vi "amplitude modulation and demodulation.vi"() -> ()   [LabVIEW 2018]
uses:
  <vilib>/express/express analysis/Spectral/Block/exnSpectralBlock spectral measurements RMS poly.vi
  <vilib>/express/express analysis/Spectral/Block/exnSpectralBlock spectral measurements RMS DDT.vi
  <vilib>/express/express analysis/Spectral/XNode/ExpressSpectralMeasurementsBlockNode.xnode
panel:
  out "Waveform Graph 3":dynamicdata(graph)
  out "Waveform Graph 2":dynamicdata(graph)
  in  "Numeric 3":dbl
  out "Waveform Graph":dynamicdata(graph)
  in  "stop":bool
  in  "Numeric 2":dbl
  in  "Numeric":dbl
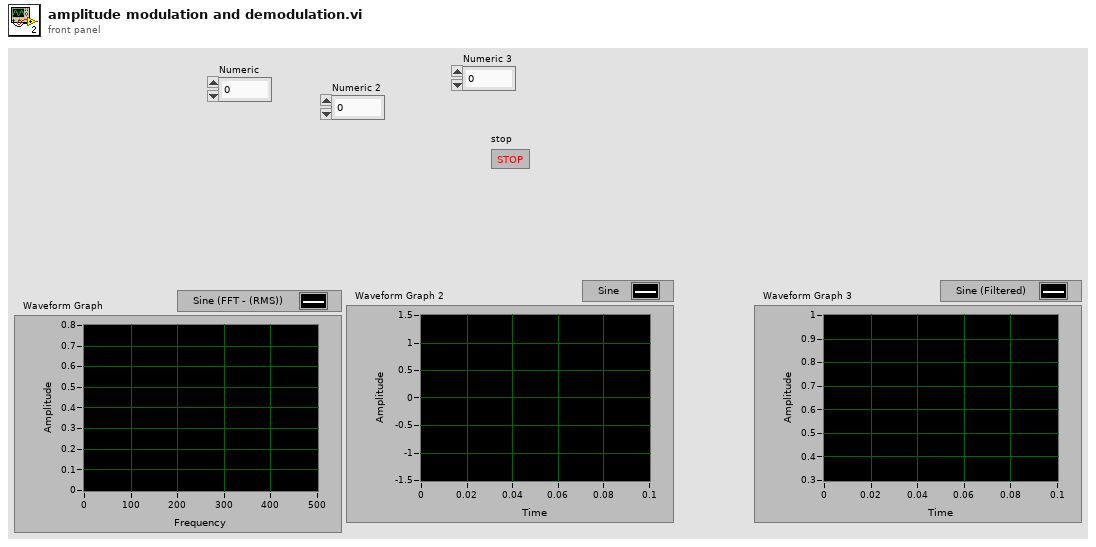
[diagram p1: front panel]
types:
  T1 = cluster{"averaging mode":u16, "weighting mode":u16, "number of averages":u32}
  T2 = cluster{"dB On (F)":bool, "unwrap phase (F)":bool, "convert to degree (F)":bool}
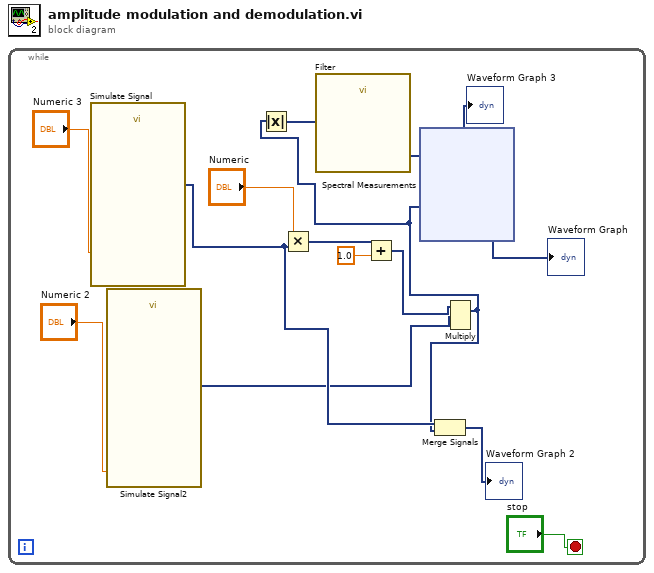
[diagram p0: block diagram]
diagram:
  n1 = while {
    stop <- "stop" stop-if-true
    n2 = call "Simulate Signal"("Frequency"="Numeric 3") -> ("Sine"=w7:dynamicdata)  [unwired: 13 in, 1 out]
    n3 = call "Simulate Signal2"("Frequency"="Numeric 2") -> ("Sine"=w5:dynamicdata)  [unwired: 13 in, 1 out]
    n4 = Multiply(x="Numeric", y=w7) -> (x*y=w13:dynamicdata)
    n5 = Add(x=w13, y=1.0) -> (x+y=w4:dynamicdata)
    n6 = Multiply(1:w5, 2:w4) -> (0:w2:dynamicdata)  [unwired: 1 in, 1 out]
    n7 = Absolute Value(x=w2) -> (abs(x)=w3:dynamicdata)
    n8 = call "Filter"("Signal"=w3) -> ("Filtered Signal"=→"Waveform Graph 3":dynamicdata)  [unwired: 9 in, 1 out]
    n9 = xnode "Spectral Measurements"("Signals"=w2) -> ("FFT - (RMS)"=→"Waveform Graph":dynamicdata)  [unwired: 1 in, 2 out]
    n10 = Merge Signals(w7, w2) -> (→"Waveform Graph 2":dynamicdata)
  }
